vi "half adder 2.vi"(10 "Boolean 3":bool, 11 "Cin":bool) -> (2 "Boolean":bool, 3 "Boolean 2":bool)   [LabVIEW 2018]
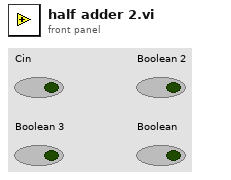
[diagram p1: front panel]
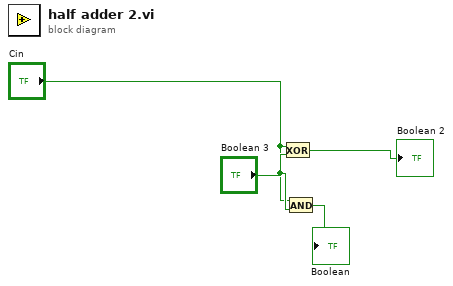
[diagram p0: block diagram]
diagram:
  n1 = Exclusive Or(1:"Boolean 3", 2:"Cin") -> (0:→"Boolean 2":bool)
  n2 = And(x="Cin", y="Boolean 3") -> (x .and. y?=→"Boolean":bool)
